vi "Shutdown.vi"(8 "error in":errorcluster, 11 "Network Protocol in":refnum<class "Network Protocol.lvclass">) -> (0 "error out":errorcluster)   [LabVIEW 2021, in "Network Protocol.lvclass"]
doc: "This provides an interface for the master to open a connection to the slave."
uses:
  Network Protocol.lvclass
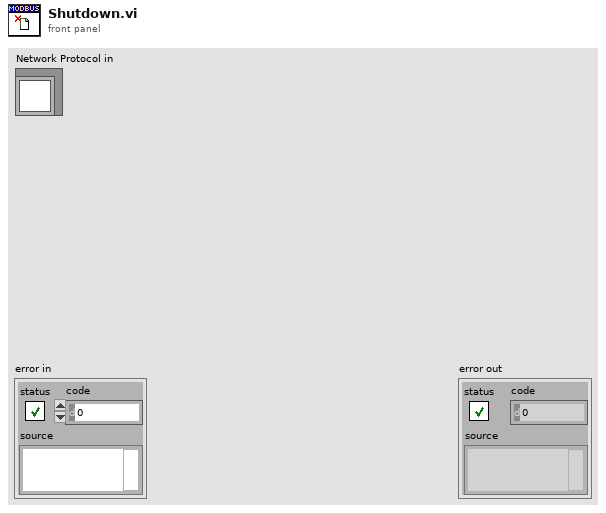
[diagram p1: front panel]
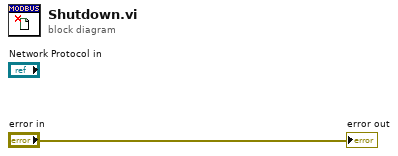
[diagram p0: block diagram]
diagram:
  "error out" <- "error in"
